vi "libssh2_knownhost_init.vi"(8 "error in (no error)":errorcluster, 11 "session":T1) -> (0 "error out":errorcluster, 3 "known hosts collection":T2)   [LabVIEW 2013, in "libssh2.lvlib"]
doc: "Initializes a collection of known hosts for this session."
uses:
  libssh2.lvlib
  Known Hosts Collection Refnum.ctl
  Session Refnum.ctl
  Global Settings.vi
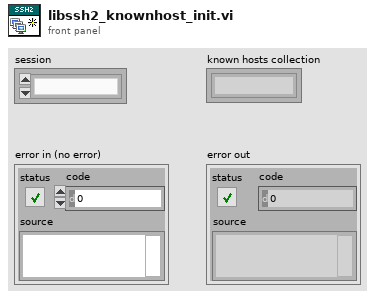
[diagram p1: front panel]
types:
  T1 = typedef "libssh2.lvlib/Session Refnum.ctl" = refnum<k1>
  T2 = typedef "libssh2.lvlib/Known Hosts Collection Refnum.ctl" = refnum<k1>
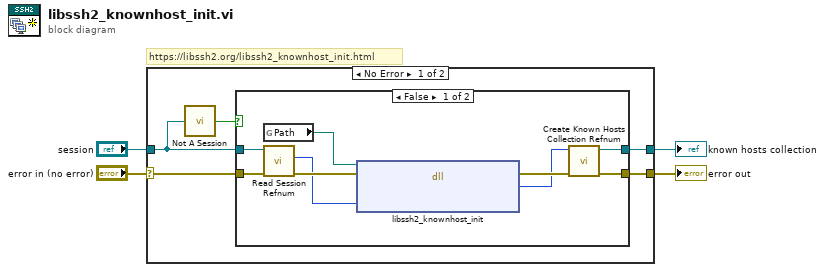
[diagram p0: block diagram]
diagram:
  # "https://libssh2.org/libssh2_knownhost_init.html"
  n1 = case shown="No Error" "error in (no error)" {
    selector: "error in (no error)" -> [w7 w20]
    tunnel: "session" -> [w5 _]
    tunnel: [w9 w20] -> w3
    tunnel: [w8 _] -> w2
    frame No Error {
      n2 = call "Not A Session.vi"("session"=w5) -> ("Not a Session?"=w6:bool)
      n3 = case shown="False" w6 {
        tunnel: w5 -> [w16 _]
        tunnel: [w14 w19] -> w9
        tunnel: [w12 _] -> w8
        tunnel: w7 -> [w11 w19]
        frame False {
          n4 = global read "Global Settings.vi" "Path"() -> (w10:path)
          n5 = call "Read Session Refnum.vi"("error in (no error)"=w11, "session"=w16) -> ("error out"=w17:errorcluster, "LIBSSH2_SESSION*"=w15:u64)  [unwired: 8 in]
          n6 = dll-call lib="C:/Users/pasca/source/repos/libssh2-labview/libssh2/libssh2**.*" fn="libssh2_knownhost_init"(path in=w10, error in=w17, "session"=w15) -> (error out=w18:errorcluster, "return value"=w13:u64)  [unwired: 2 in, 1 out]
          n7 = call "Create Known Hosts Collection Refnum.vi"("error in (no error)"=w18, "LIBSSH2_KNOWNHOSTS*"=w13) -> ("error out"=w14:errorcluster, "known hosts collection"=w12:T2)  [unwired: 8 in]
        }
        frame True {
        }
      }
    }
    frame Error {
    }
  }
  "known hosts collection" <- w2
  "error out" <- w3
